vi "My Custom Controls - Node Browser.vi"() -> ()   [LabVIEW 2016]
doc: "Sample numeric display item."
uses:
  <vilib>/NI Veristand/Display Template Support/Display Template Support.llb/enum_Display Template Handler Minimal To Widget Msg.ctl
  <vilib>/NI Veristand/Display Template Support/Display Template Support.llb/enum_Display Template Handler Minimal To Workspace.ctl
  <vilib>/NI Veristand/Execution/Workspace/NI_VS Workspace ExecutionAPI.lvlib
  <vilib>/NI Veristand/Display Template Support/Display Template Support.llb/sub_Display Template Handler Custom.vi
  NationalInstruments.VeriStand.SystemStorageUI
  <vilib>/NI Veristand/UI Controls/Single Node Browser/NI_VS UI Single Node Browser.lvlib
  NationalInstruments.VeriStand.SystemStorage
  <vilib>/NI Veristand/Display Template Support/Display Template Support.llb/cluster_Screen Item Settings.ctl
  <vilib>/NI Veristand/Display Template Support/Display Template Support.llb/cluster_Graph Scale Settings.ctl
  <vilib>/NI Veristand/Display Template Support/Display Template Support.llb/cluster_Graph Plot Settings.ctl
panel:
  in  "Tree Browser":refnum<k24>(container)
  in  "Single Node Browser":refnum<k24>(container)
  in  "NIVS.System Definition Root":refnum<k24>
  in  "NIVS.Gateway IP Address":string
  in  "Message Display":string
  in  "Item.Data":T1
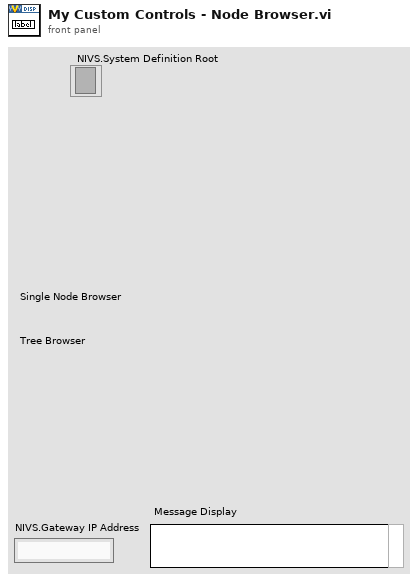
[diagram p1: front panel]
types:
  T1 = typedef "cluster_Screen Item Settings.ctl" = cluster{"Template VI":string, "Position X":i32, "Position Y":i32, "Custom":string, "Show Title Bar":bool, "ID":i32, "Always On Top":bool, "Allow Resize":bool, "Allow Minimize":bool, "Allow Close":bool, "Size to Screen":bool, "Screen.ID":i32, "State":enum16{"Normal", "New"}, "Title":string, "Window Bounds":cluster{"[0]":i16, "[1]":i16, "[2]":i16, "[3]":i16}, "Channel Ref":u64, "Unit":string, "Default Units?":bool, "Flash Limit?":bool, "Color 1":u32, "Color 2":u32, "Color 3":u32, "Color 4":u32, "Bck Color":u32, "Fore Color":u32, "Limit 1":dbl, "Limit 2":dbl, "Limit 3":dbl, "Limit 4":dbl, "Limit Mode 1":i32, "Limit Mode 2":i32, "Limit Mode 3":i32, "Limit Mode 4":i32, "Scale Precision":i32, "Scale Min":dbl, "Scale Max":dbl, "Format":i32, "Precision":i32, "Background Type":i32, "IDs":i32[], "Units":string[], "Labels":string[], "Scale Factor":dbl, "Scale Offset":dbl, "YScale Index":u32[], "XScale":T2, "YScales":T2[], "Plots":T3[], "Update Period":dbl, "History Length":dbl, "My.Ref":refnum<vi>, "Is Control?":bool, "Channel Paths":string[], "Custom Data":variant}
  T2 = typedef "cluster_Graph Scale Settings.ctl" = cluster{"Format":u8, "Precision":u8, "Fit":u8, "Label":string, "Use Default Label":bool, "Label Visible":bool, "Min":dbl, "Max":dbl}
  T3 = typedef "cluster_Graph Plot Settings.ctl" = cluster{"Bar Style":u8, "Fill To":i16, "Fill/PtColor":u32, "Line Style":u8, "Line Width":u8, "Color":u32, "Interp":u8, "Point Style":u8}
  T4 = typedef "enum_Display Template Handler Minimal To Workspace.ctl" = cluster{"Operation":enum16{"SetCustomData", "DeleteItem"}, "Data":variant}
  T5 = typedef "enum_Display Template Handler Minimal To Widget Msg.ctl" = enum16{"Stop", "LaunchConfigDialog"}
  T6 = typedef "NI_VS UI Single Node Browser.lvlib/Callback Type.ctl" = cluster{"Net Callbacks":refnum<k27>[], "Event":refnum<user-event>}
  T7 = typedef "NI_VS Workspace ExecutionAPI.lvlib/WorkspaceAPI.ctl" = refnum<k24>
  T8 = typedef "NI_VS Workspace ExecutionAPI.lvlib/SystemStateEventRef.ctl" = cluster{"CustDatRef":refnum<user-event>, "EvtRef":refnum<k27>, "Target State User Event":refnum<user-event>}
  T9 = typedef "NI_VS Workspace ExecutionAPI.lvlib/SystemStateRegEventRef.ctl" = refnum<event-registration>
  T10 = cluster{"Event Registration Refnum":refnum<event-registration>, "SystemChangeEventRef":T9}
  T11 = typedef "NI_VS UI Single Node Browser.lvlib/Node Ref.ctl" = refnum<k24>
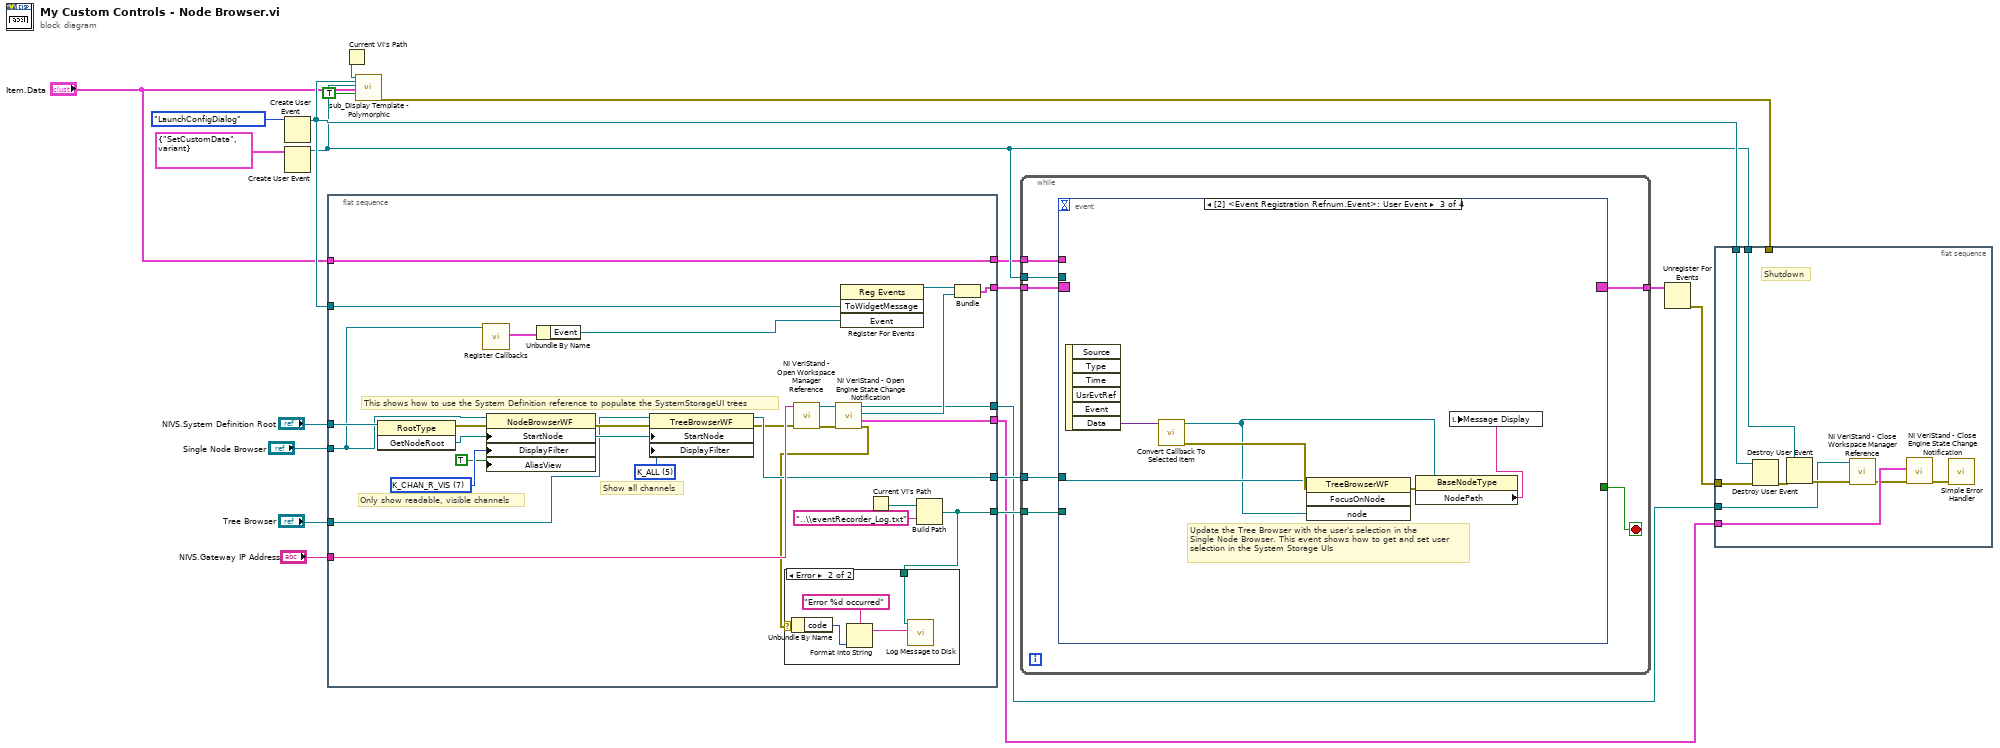
[diagram p0: block diagram]
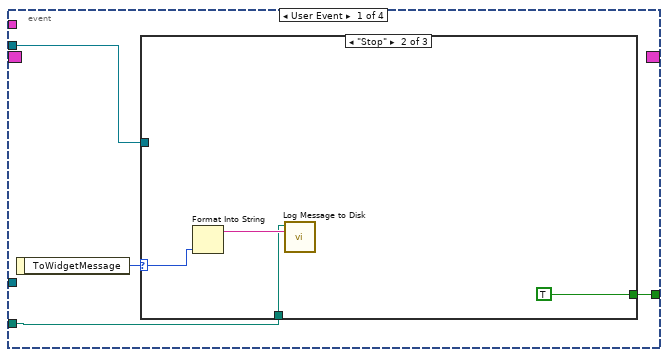
[diagram p3: hidden frame]
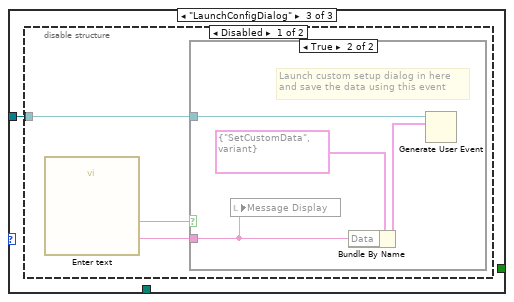
[diagram p5: hidden frame]
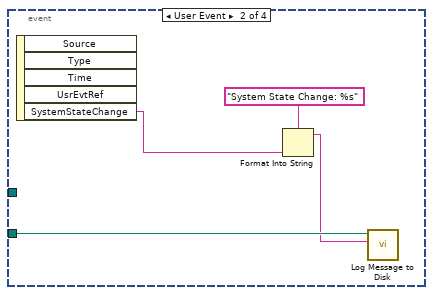
[diagram p8: hidden frame]
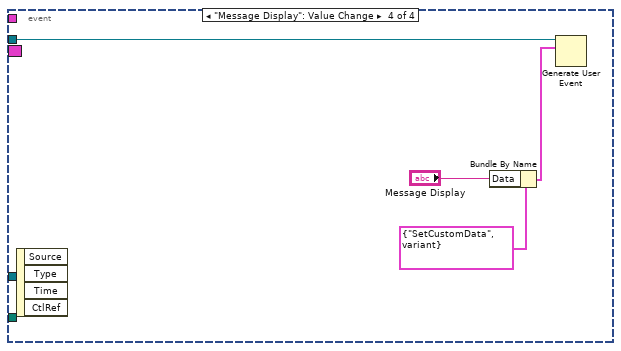
[diagram p9: hidden frame]
diagram:
  n1 = Create User Event(user event datatype=enum_Display_Template_Handler_Minimal_To_Widget_Msg."LaunchConfigDialog" ("ToWidgetMessage")) -> (user event=w16:refnum<user-event>)  [unwired: 1 in, 1 out]
  n2 = Create User Event(user event datatype=T4 {"Operation"=enum."SetCustomData", "Data"=variant} ("Data")) -> (user event=w12:refnum<user-event>)  [unwired: 1 in, 1 out]
  n3 = flat-sequence {
    tunnel: [w45] -> w18
    tunnel: w16 -> [w47]
    tunnel: "Item.Data" -> [w44]
    tunnel: [w44] -> w10
    tunnel: "NIVS.System Definition Root" -> [w33]
    tunnel: "Single Node Browser" -> [w31]
    tunnel: "Tree Browser" -> [w32]
    tunnel: "NIVS.Gateway IP Address" -> [w28]
    tunnel: [w27] -> w5
    tunnel: [w23] -> w4
    tunnel: [w22] -> w2
    tunnel: [w21] -> w1
    frame #0 {
      w37 = u8 7 items=["K_CHAN_R", "K_CHAN_W", "K_CHAN_RW", "K_CHAN_VOLT", "K_CHAN_FAULT", "K_ALL", "K_CUSTOM", "K_CHAN_R_VIS", "K_CHAN_W_VIS", "K_CHAN_RW_VIS", "K_CHAN_VOLT_VIS", "K_CHAN_FAULT_VIS"] ("DisplayFilter")
      w38 = u8 5 items=["K_CHAN_R", "K_CHAN_W", "K_CHAN_RW", "K_CHAN_VOLT", "K_CHAN_FAULT", "K_ALL", "K_CUSTOM", "K_CHAN_R_VIS", "K_CHAN_W_VIS", "K_CHAN_RW_VIS", "K_CHAN_VOLT_VIS", "K_CHAN_FAULT_VIS"] ("DisplayFilter")
      # "Show all channels"
      # "Only show readable, visible channels"
      # "This shows how to use the System Definition reference to populate the SystemStorageUI trees"
      n4 = invoke class="RootType" method="GetNodeRoot"(reference=w33) -> (error out=w39:errorcluster, "GetNodeRoot"=w40:refnum<k24>)  [unwired: 2 in, 1 out]
      n5 = call <vilib>:"Register Callbacks.vi"("Single Node Browser"=w31) -> ("Callbacks"=w43:T6)  [unwired: 8 in, 2 out]
      n6 = property class="NodeBrowserWF"(reference=w31, error in=w39, "StartNode"=w40, "DisplayFilter"=w37, "AliasView"=TRUE) -> (error out=w41:errorcluster)  [unwired: 1 out]
      n7 = Unbundle By Name(w43) -> ("Event"=w42:refnum<user-event>)
      n8 = property class="TreeBrowserWF"(reference=w32, error in=w41, "StartNode"=w40, "DisplayFilter"=w38) -> (reference out=w27:refnum<k24>, error out=w25:errorcluster)
      n9 = call <vilib>:"NI VeriStand - Open Workspace Manager Reference.vi"("error in (no error)"=w25, "Gateway IP Address (\"\": localhost)"=w28) -> ("error out"=w30:errorcluster, "WorkspaceManager"=w29:T7)  [unwired: 8 in]
      n10 = call <vilib>:"NI VeriStand - Open Engine State Change Notification.vi"("error in (no error)"=w30, "WorkspaceManager in"=w29) -> ("error out"=w24:errorcluster, "SystemStateRefs"=w22:T8, "SystemChangeEventRef"=w26:T9, "WorkspaceManager out"=w21:T7)  [unwired: 6 in]
      n11 = register-events(w47, w42) -> (reference out=w46:refnum<event-registration>)  [unwired: 2 in, 1 out]
      n12 = Current VI's Path() -> (path=w34:path)
      n13 = Build Path(base path=w34, name or relative path="..\\eventRecorder_Log.txt") -> (appended path=w23:path)
      n14 = case shown="Error" w24 {
        selector: w24 -> [_ w52]
        tunnel: w23 -> [_ w48]
        frame No Error {
        }
        frame Error {
          n15 = Unbundle By Name(w52) -> ("code"=w50:i32)
          n16 = Format Into String(format string="Error %d occurred", w50) -> (resulting string=w51:string)  [unwired: 2 in, 1 out]
          n17 = call <userlib>:"Log Message to Disk.vi"("Message"=w51, "Log File Path (FM_debug.txt)"=w48) -> ()  [unwired: 9 in, 1 out]
        }
      }
      n18 = Bundle("Event Registration Refnum"=w46, "SystemChangeEventRef"=w26) -> (w45:T10)  [unwired: 1 in]
    }
  }
  n19 = Current VI's Path() -> (path=w14:path)
  n20 = call-poly <vilib>:"sub_Display Template - Polymorphic.vi"("Parent.Path"=w14, "ToWidgetEvent"=w16, "ToWorkspace"=w12, "Item.Data"="Item.Data", "Resizable"=TRUE) -> ("error out"=w20:errorcluster)  [unwired: 1 in, 13 out]
  n21 = while {
    tunnel: w18 -> [w53]
    tunnel: [w58] -> w3
    tunnel: w12 -> [w57]
    tunnel: w10 -> [w56]
    tunnel: w5 -> [w55]
    tunnel: w4 -> [w54]
    stop <- w59 stop-if-true
    n22 = event shown="[2] <Event Registration Refnum.Event>: User Event" {
      selector: w53 -> [_ _ _ _]
      dyn-events: [_ _ _ _] -> w58
      timeout: _ -> [_ _ _ _]
      tunnel: [w62 _ _ _] -> w59
      tunnel: w57 -> [w61 _ _ w89]
      tunnel: w56 -> [_ _ _ _]
      tunnel: w55 -> [_ _ w83 _]
      tunnel: w54 -> [w60 w78 _ _]
      event User Event {
        n23 = event-data() -> ("ToWidgetMessage"=w63:T5)  [unwired: 1 out]
        n24 = case shown="\"Stop\"" w63 {
          selector: w63 -> [_ w66 _]
          tunnel: [_ TRUE _] -> w62
          tunnel: w61 -> [_ _ w68]
          tunnel: w60 -> [_ w64 _]
          frame Default {
          }
          frame "Stop" {
            n25 = Format Into String(w66) -> (resulting string=w65:string)  [unwired: 3 in, 1 out]
            n26 = call <userlib>:"Log Message to Disk.vi"("Message"=w65, "Log File Path (FM_debug.txt)"=w64) -> ()  [unwired: 9 in, 1 out]
          }
          frame "LaunchConfigDialog" {
            n27 = disable-structure shown="Disabled" {
              disable-tunnel: w68 -> [w71 _]
              frame Disabled {
                n28 = call "Enter text"() -> ("Text"=w69:string, "OK"=w70:bool)  [unwired: 17 in, 1 out]
                n29 = case shown="True" w70 {
                  tunnel: w71 -> [_ w75]
                  tunnel: w69 -> [_ w72]
                  frame False {
                  }
                  frame True {
                    # "Launch custom setup dialog in here\nand save the data using this event"
                    n30 = local write "Message Display"(w72) -> ()
                    n31 = Bundle By Name(cluster=T4 {"Operation"=enum."SetCustomData", "Data"=variant} ("event data"), "Data"=w72) -> (w73:T4)
                    n32 = Generate User Event(user event=w75, event data cluster=w73) -> ()  [unwired: 2 in, 2 out]
                  }
                }
              }
              frame Enabled {
              }
            }
          }
        }
      }
      event User Event {
        n33 = event-data() -> ("SystemStateChange"=w77:string)  [unwired: 5 out]
        n34 = Format Into String(format string="System State Change: %s", w77) -> (resulting string=w76:string)  [unwired: 2 in, 1 out]
        n35 = call <userlib>:"Log Message to Disk.vi"("Message"=w76, "Log File Path (FM_debug.txt)"=w78) -> ()  [unwired: 9 in, 1 out]
      }
      event User Event {
        # "Update the Tree Browser with the user's selection in the\nSingle Node Browser. This event shows how to get and set user\nselection in the System Storage UIs"
        n36 = event-data() -> ("Data"=w84:variant)  [unwired: 6 out]
        n37 = call <vilib>:"Convert Callback To Selected Item.vi"("Data"=w84) -> ("error out"=w85:errorcluster, "Selected Item"=w81:T11)  [unwired: 9 in]
        n38 = invoke class="TreeBrowserWF" method="FocusOnNode"(reference=w83, error in=w85, "node"=w81) -> (error out=w82:errorcluster)  [unwired: 1 in, 3 out]
        n39 = property class="BaseNodeType"(reference=w81, error in=w82) -> ("NodePath"=w80:string)  [unwired: 2 out]
        n40 = local write "Message Display"(w80) -> ()
      }
      event "Message Display": Value Change {
        n41 = event-data() -> ()  [unwired: 5 out]
        n42 = Bundle By Name(cluster=T4 {"Operation"=enum."SetCustomData", "Data"=variant} ("event data"), "Data"="Message Display") -> (w86:T4)
        n43 = Generate User Event(user event=w89, event data cluster=w86) -> ()  [unwired: 2 in, 2 out]
      }
    }
  }
  n44 = Unregister For Events(event registration refnum=w3) -> (error out=w17:errorcluster)  [unwired: 1 in]
  n45 = flat-sequence {
    tunnel: w20 -> [_]
    tunnel: w17 -> [w97]
    tunnel: w16 -> [w98]
    tunnel: w12 -> [w95]
    tunnel: w2 -> [w92]
    tunnel: w1 -> [w93]
    frame #0 {
      # "Shutdown"
      n46 = Destroy User Event(user event=w98, error in=w97) -> (error out=w96:errorcluster)
      n47 = Destroy User Event(user event=w95, error in=w96) -> (error out=w94:errorcluster)
      n48 = call <vilib>:"NI VeriStand - Close Workspace Manager Reference.vi"("error in (no error)"=w94, "WorkspaceManager"=w93) -> ("error out"=w91:errorcluster)  [unwired: 9 in]
      n49 = call <vilib>:"NI VeriStand - Close Engine State Change Notification.vi"("error in (no error)"=w91, "SystemStateRefs"=w92) -> ("error out"=w90:errorcluster)  [unwired: 9 in]
      n50 = call <vilib>:"Simple Error Handler.vi"("error in (no error)"=w90) -> ()  [unwired: 4 in, 5 out]
    }
  }
